vi "FlatToRichcif_manager_QueryPluginTypesRequest.vi"(5 "OutputClusterType":T1, 11 "InputCluster":T2) -> (3 "OutputCluster":T1)   [LabVIEW 2021, in "CIF_Manager_client.lvlib"]
uses:
  cif_manager_QueryPluginTypesRequest_Flat.ctl
  cif_manager_QueryPluginTypesRequest.ctl
  CIF_Manager_client.lvlib
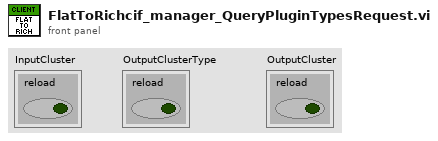
[diagram p1: front panel]
types:
  T1 = typedef "CIF_Manager_client.lvlib/cif_manager_QueryPluginTypesRequest.ctl" = cluster{"reload":bool}
  T2 = typedef "CIF_Manager_client.lvlib/cif_manager_QueryPluginTypesRequest_Flat.ctl" = cluster{"reload":bool}
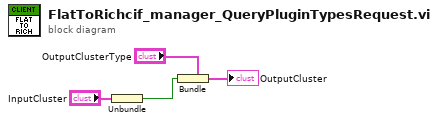
[diagram p0: block diagram]
diagram:
  n1 = Unbundle "Unbundle"("InputCluster") -> ("reload"=w1:bool)
  n2 = Bundle "Bundle"(cluster="OutputClusterType", "reload"=w1) -> (→"OutputCluster":T1)
